vi "Test_TimeoutStop_NoLastMessage_LastMessageNotExecuted.vi"(8 "error in (no error)":errorcluster, 11 "TestCase in":refnum<class "TestMessageCycle.lvclass">) -> (0 "error out":errorcluster, 3 "TestCase out":refnum<class "TestMessageCycle.lvclass">)   [LabVIEW 2017, in "TestMessageCycle.lvclass"]
uses:
  TestMessageCycle.lvclass
  <vilib>/ActorFramework/Message/Message.lvclass
  Source/MessageCycle/Message Cycle Notifications.ctl
  Source/MessageCycle/MessageCycle.lvclass/MessageCycle.ctl
  <vilib>/ActorFramework/Message Enqueuer/Message Enqueuer.lvclass/Message Enqueuer.ctl
  1b07eade-a78c-42fd-a35c-617bb70b86e5.vi
  <vilib>/ActorFramework/Message Enqueuer/Enqueue.vi
  Doubles/MessageCountsExecutions/MessageCountsExecutions.lvclass
  C:/Program Files (x86)/National Instruments/LabVIEW 2017/vi.lib/ActorFramework/Message/Message.lvclass
  Doubles/ActorCountsMessageCycles/ActorCountsMessageCycles.lvclass
  C:/Program Files (x86)/National Instruments/LabVIEW 2017/vi.lib/ActorFramework/Actor/Actor.lvclass
  Source/MessageCycle/MessageCycle.lvclass
  <vilib>/ActorFramework/Stop Msg/Stop Msg.lvclass
  Source/MessageCycle/Launch Deferred Timeout Notifier.vi
  <vilib>/ActorFramework/Message Priority Queue/Priority Enqueue.vi
  <vilib>/ActorFramework/Actor/Actor.lvclass
panel:
  out "\"Last Message\" Executions":u32
  out "Cyclic Messages Received":u32
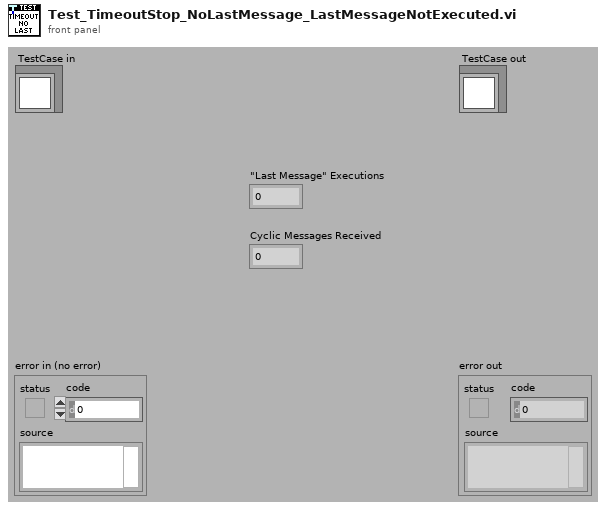
[diagram p1: front panel]
types:
  T1 = typedef "MessageCycle.lvclass/Message Cycle Notifications.ctl" = enum16{"Process Final Copy and Stop", "Stop Immediately", "Substitute Last Message and Stop"}
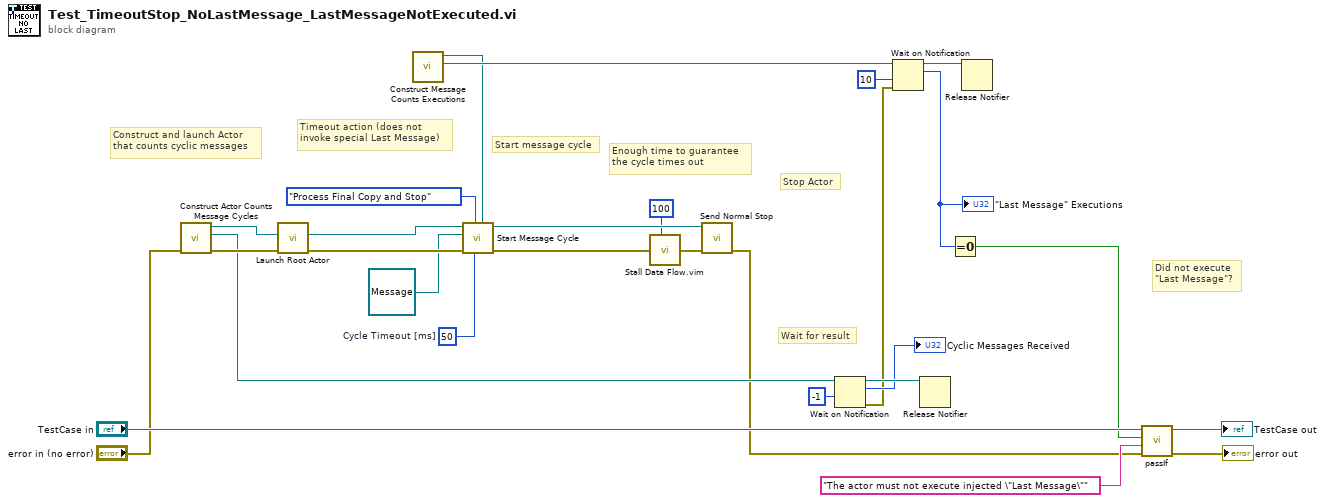
[diagram p0: block diagram]
diagram:
  w3 = 50  # Cycle Timeout [ms]
  # "Enough time to guarantee\nthe cycle times out"
  # "Timeout action (does not\ninvoke special Last Message)"
  # "Wait for result"
  # "Stop Actor"
  # "Start message cycle"
  # "Did not execute\n\"Last Message\"?"
  # "Construct and launch Actor\nthat counts cyclic messages"
  n1 = call "Construct Actor Counts Message Cycles.vi"("error in (no error)"="error in (no error)") -> ("error out"=w18:errorcluster, "Final Count"=w17:refnum<notifier>, "ActorCountsMessageCycles"=w20:refnum<class "ActorCountsMessageCycles.lvclass">)  [unwired: 8 in]
  n2 = call <vilib>:"Launch Root Actor.vi"("error in (no error)"=w18, "Actor"=w20) -> ("error out"=w28:errorcluster, "Actor's Enqueuer"=w24:refnum<class "Message Enqueuer.lvclass">)  [unwired: 8 in]
  n3 = call "Construct Message Counts Executions.vi"() -> ("Message Executions"=w7:refnum<notifier>, "CyclicMessageCountsCycles out"=w1:refnum<class "MessageCountsExecutions.lvclass">)  [unwired: 9 in, 1 out]
  n4 = call "Start Message Cycle.vi"("Last Message"=w1, "Cycle Timeout [ms] (-1)"=w3, "Timeout Action"=Message_Cycle_Notifications."Process Final Copy and Stop", "error in (no error)"=w28, "Message"=refnum<class "Message.lvclass"> refnum, "Message Enqueuer"=w24) -> ("error out"=w12:errorcluster, "Message Enqueuer out"=w23:refnum<class "Message Enqueuer.lvclass">)  [unwired: 3 in, 1 out]
  n5 = call "Stall Data Flow.vim"("value in"=w12, "milliseconds to wait"=u32 100) -> ("value out"=w11:errorcluster)  [unwired: 1 out]
  n6 = call <vilib>:"Send Normal Stop.vi"("error in (no error)"=w11, "Message Enqueuer"=w23) -> ("error out"=w14:errorcluster)  [unwired: 9 in]
  n7 = Wait on Notification(notifier=w17, timeout in ms (-1)=-1) -> (notifier out=w15:refnum<notifier>, notification=→"Cyclic Messages Received":u32, error out=w8:errorcluster)  [unwired: 2 in, 1 out]
  n8 = Wait on Notification(notifier=w7, timeout in ms (-1)=10, error in (no error)=w8) -> (notifier out=w6:refnum<notifier>, notification=w5:u32)  [unwired: 1 in, 2 out]
  "\"Last Message\" Executions" <- w5
  n9 = Release Notifier(notifier=w15) -> ()  [unwired: 2 in, 3 out]
  n10 = Equal To 0?(x=w5) -> (x = 0?=w22:bool)
  n11 = Release Notifier(notifier=w6) -> ()  [unwired: 2 in, 3 out]
  n12 = call-dynamic "passIf.vi"("error in (no error)"=w14, "message (\"\")"="The actor must not execute injected \"Last Message\"" ("message (\"\")"), "pass"=w22, "TestCase in"="TestCase in") -> ("error out"=→"error out":errorcluster, "TestCase out"=→"TestCase out":refnum<class "TestMessageCycle.lvclass">)  [unwired: 6 in]
